vi "XIPIN_SelectIO_Interface_Wizard_5_1.vi"   [LabVIEW 2017]
doc: "The SelectIO Interface Wizard creates a HDL file (Verilog or VHDL) that contains IO logic such as SERDES and IODELAY blocks customized to the user's interface requirements.\n------------------------------------\n<b>Need License</b> : No"
uses:
  <vilib>/rvi/XilinxIP/XIPIN_XNode/niFpgaXIPIN.xnode
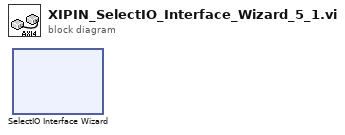
[diagram p0: block diagram]
diagram:
  n1 = xnode ("SelectIO Interface Wizard")() -> ()
